vi "Update Errors and Info.vi"(8 "error in (no error)":errorcluster, 9 "Get All Info":bool, 10 "Get All Errors":bool, 11 "CIF_UI in":refnum<class "CIF_UI.lvclass">) -> (0 "error out":errorcluster, 1 "Info":string, 2 "Error Count":i32, 3 "CIF_UI out":refnum<class "CIF_UI.lvclass">)   [LabVIEW 2021, in "CIF_UI.lvclass"]
uses:
  CIF_UI.lvclass
  CIF_UI.lvclass/CIF_UI.ctl
  CIFPluginManager/CIFPluginManager/gRPC/CIF_Manager_Client_Wrapper/CIFManagerClientWrapper.lvlib
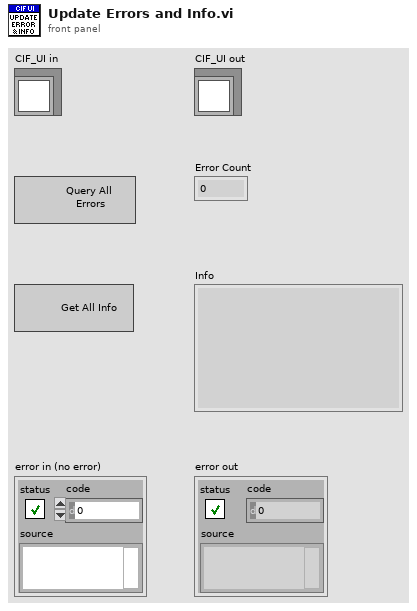
[diagram p1: front panel]
types:
  T1 = typedef "grpc-lvsupport-release.lvlib/grpcId.ctl" = u64
  T2 = typedef "CIF_Manager_client.lvlib/cif_manager_ErrorInfo.ctl" = cluster{"error_status":bool, "error_code":i32, "plugin":string, "time":string, "message":string, "location":string}
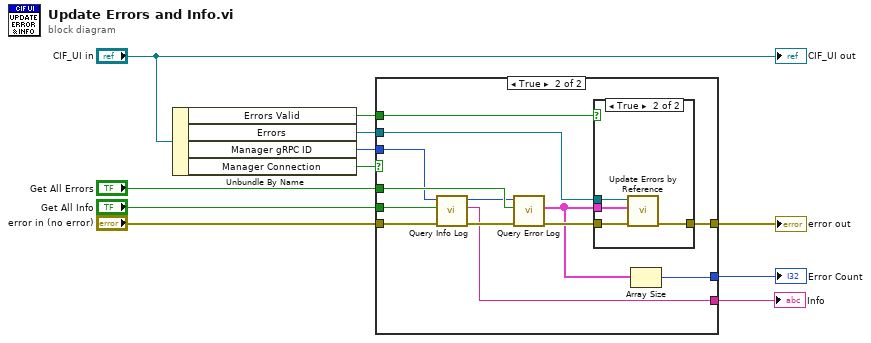
[diagram p0: block diagram]
diagram:
  n1 = Unbundle By Name("CIF_UI in") -> ("Errors Valid"=w1:bool, "Errors"=w8:refnum<vi>, "Manager gRPC ID"=w4:T1, "Manager Connection"=w2:bool)
  n2 = case shown="True" w2 {
    tunnel: "Get All Errors" -> [_ w24]
    tunnel: "Get All Info" -> [_ w23]
    tunnel: w8 -> [_ w21]
    tunnel: [w12 w18] -> w7
    tunnel: [_ w17] -> w6
    tunnel: [_ w16] -> w5
    tunnel: w4 -> [_ w15]
    tunnel: "error in (no error)" -> [w12 w14]
    tunnel: w1 -> [_ w13]
    frame False {
    }
    frame True {
      n3 = call "Query Info Log.vi"("error in"=w14, "query_all"=w23, "gRPC ID in"=w15) -> ("error out"=w19:errorcluster, "Info"=w16:string, "gRPC ID out"=w20:T1)  [unwired: 6 in]
      n4 = call "Query Error Log.vi"("error in"=w19, "query_all"=w24, "gRPC ID in"=w20) -> ("error out"=w25:errorcluster, "error_info"=w22:T2[])  [unwired: 6 in, 1 out]
      n5 = case shown="True" w13 {
        tunnel: w25 -> [w26 w30]
        tunnel: w22 -> [_ w29]
        tunnel: w21 -> [_ w28]
        tunnel: [w26 w27] -> w18
        frame False {
        }
        frame True {
          n6 = call "Update Errors by Reference.vi"("error in (no error)"=w30, "error_info"=w29, "Error MCLB reference in"=w28) -> ("error out"=w27:errorcluster)  [unwired: 7 in, 1 out]
        }
      }
      n7 = Array Size(array=w22) -> (size(s)=w17:i32)
    }
  }
  "error out" <- w7
  "Error Count" <- w6
  "Info" <- w5
  "CIF_UI out" <- "CIF_UI in"
